vi "Update Temperature and Setpoint Graph.vi"(1 "Temp and SetPoint":dbl[](array[numeric])) -> (0 "error out":errorcluster)   [LabVIEW 2011]
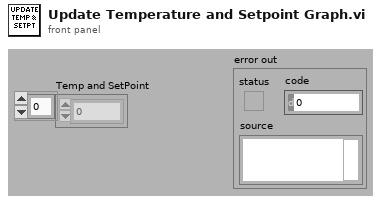
[diagram p1: front panel]
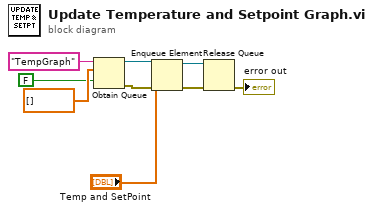
[diagram p0: block diagram]
diagram:
  n1 = Obtain Queue(name (unnamed)="TempGraph", element data type=dbl[] [], create if not found? (T)=FALSE) -> (queue out=w7:refnum<queue>, error out=w5:errorcluster)  [unwired: 2 in, 1 out]
  n2 = Enqueue Element(queue=w7, element="Temp and SetPoint", error in (no error)=w5) -> (queue out=w2:refnum<queue>, error out=w3:errorcluster)  [unwired: 2 out]
  n3 = Release Queue(queue=w2, error in (no error)=w3) -> (error out=→"error out":errorcluster)  [unwired: 3 out]
